vi "Create Message Paths.vi"(6 "Message":T1, 8 "error in (no error)":errorcluster, 11 "LV-Protoc in":refnum<class "LV-Protoc.lvclass">) -> (0 "error out":errorcluster, 3 "LV-Protoc out":refnum<class "LV-Protoc.lvclass">, 4 "Message Paths":T5)   [LabVIEW 2020, in "LV-Protoc.lvlib" / "LV-Protoc.lvclass"]
uses:
  LV-Protoc.lvclass
  Message Paths.ctl
  LV-Proto/Message.ctl
  LV-Proto/Field.ctl
  LV-Proto/Type.ctl
  LV-Proto/Proto Type.ctl
  LV-Protoc.lvclass/LV-Protoc.ctl
  LV-Protoc.lvlib
  LV-Proto/LV-Proto.lvlib
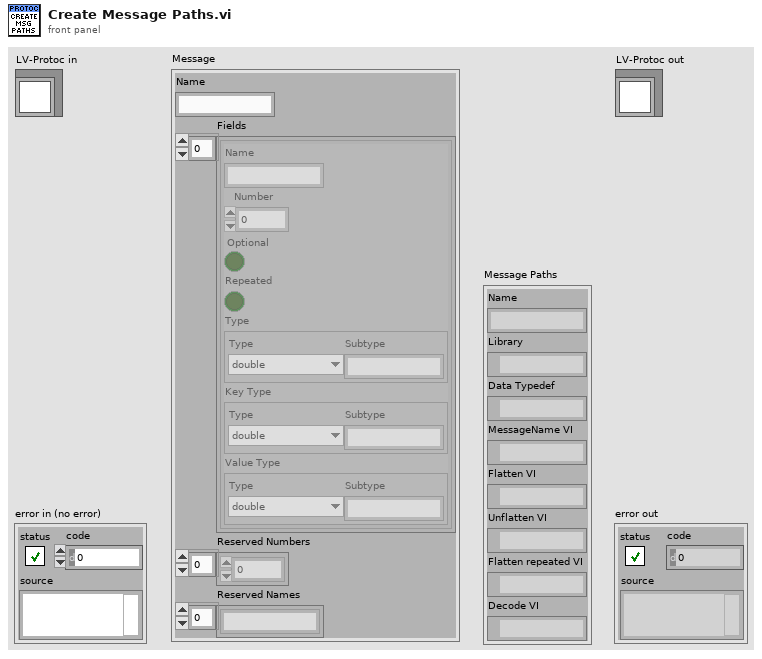
[diagram p1: front panel]
types:
  T1 = typedef "LV-Proto.lvlib/Message.ctl" = cluster{"Name":string, "Fields":T2[], "Reserved Numbers":u32[], "Reserved Names":string[]}
  T2 = typedef "LV-Proto.lvlib/Field.ctl" = cluster{"Name":string, "Number":u32, "Optional":bool, "Repeated":bool, "Type":T3, "Key Type":T3, "Value Type":T3}
  T3 = typedef "LV-Proto.lvlib/Type.ctl" = cluster{"Type":T4, "Subtype":string}
  T4 = typedef "LV-Proto.lvlib/Proto Type.ctl" = enum16{"UNKNOWN", "double", "float", "int32", "int64", "uint32", "uint64", "sint32", "sint64", "fixed32", "fixed64", "sfixed32", "sfixed64", "bool", "string", "bytes", "enum", "map", "message"}
  T5 = typedef "LV-Protoc.lvlib/Message Paths.ctl" = cluster{"Name":string, "Library":path, "Data Typedef":path, "MessageName VI":path, "Flatten VI":path, "Unflatten VI":path, "Flatten repeated VI":path, "Decode VI":path}
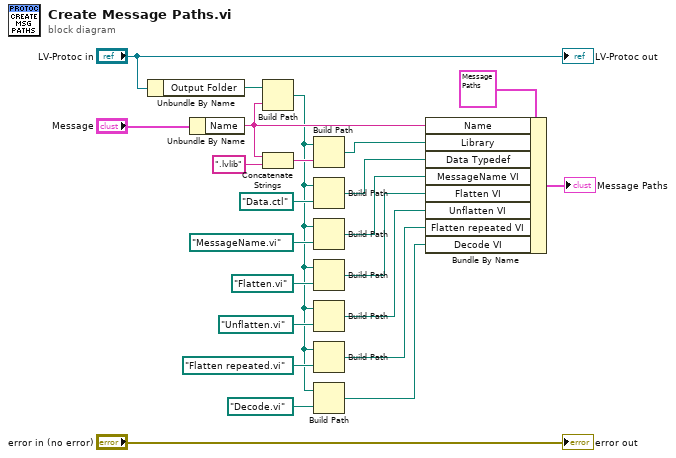
[diagram p0: block diagram]
diagram:
  n1 = Unbundle By Name("LV-Protoc in") -> ("Output Folder"=w18:path)
  n2 = Unbundle By Name("Message") -> ("Name"=w17:string)
  n3 = Build Path(base path=w18, name or relative path=w17) -> (appended path=w2:path)
  n4 = Concatenate Strings(w17, ".lvlib" ("string")) -> (w16:string)
  n5 = Build Path(base path=w2, name or relative path=w16) -> (appended path=w11:path)
  n6 = Build Path(base path=w2, name or relative path=path "Data.ctl") -> (appended path=w10:path)
  n7 = Build Path(base path=w2, name or relative path=path "MessageName.vi") -> (appended path=w9:path)
  n8 = Build Path(base path=w2, name or relative path=path "Flatten.vi") -> (appended path=w8:path)
  n9 = Build Path(base path=w2, name or relative path=path "Unflatten.vi") -> (appended path=w7:path)
  n10 = Build Path(base path=w2, name or relative path=path "Flatten repeated.vi") -> (appended path=w4:path)
  n11 = Build Path(base path=w2, name or relative path=path "Decode.vi") -> (appended path=w1:path)
  n12 = Bundle By Name(cluster=T5 {"Name"="", "Library"=path "", "Data Typedef"=path "", "MessageName VI"=path "", "Flatten VI"=path "", "Unflatten VI"=path "", "Flatten repeated VI"=path "", "Decode VI"=path ""} ("Message Paths"), "Name"=w17, "Library"=w11, "Data Typedef"=w10, "MessageName VI"=w9, "Flatten VI"=w8, "Unflatten VI"=w7, "Flatten repeated VI"=w4, "Decode VI"=w1) -> (→"Message Paths":T5)
  "error out" <- "error in (no error)"
  "LV-Protoc out" <- "LV-Protoc in"
